vi "main_cr.vi"() -> ()   [LabVIEW 2017]
panel:
  out "error out 6":errorcluster
  in  "MoveL":bool
  out "error out 5":errorcluster
  out "error out 4":errorcluster
  out "error out 3":errorcluster
  out "DigitalOutput":u8[](array[numeric])
  out "DigitalInput":u8[](array[numeric])
  out "Current SpeedFactor":dbl
  out "error out 2":errorcluster
  in  "Digital Outputs Index:":i32=1 min=1 max=16 step=1
  out "Error Log":string
  in  "GetErrorID":bool
  out "x value":string
  out "y value":string
  out "z value":string
  out "rx value":string
  out "ry value":string
  out "rz value":string
  out "j6 value":string
  out "j5 value":string
  out "j4 value":string
  out "j3 value":string
  out "j2 value":string
  out "j1 value":string
  in  "rz-":bool
  in  "ry-":bool
  in  "rx-":bool
  in  "z-":bool
  in  "y-":bool
  in  "x-":bool
  in  "rz+":bool
  in  "ry+":bool
  in  "rx+":bool
  in  "z+":bool
  in  "y+":bool
  in  "x+":bool
  in  "JointMovJ":bool
  in  "j6":dbl
  in  "j5":dbl
  in  "j4":dbl
  in  "j3":dbl
  in  "j2":dbl
  in  "j1":dbl
  in  "Set IO confrim":bool
  in  "Status":string(combo)="1"
  in  "Reset Robot":bool
  in  "Feedback Port":string="30004"
  in  "Move Port":string="30003"
  in  "Dashboard Port":string="29999"
  in  "IP Address":string="192.168.5.1"
  in  "stop get state":bool
  out "state error out 2":errorcluster
  out "Robot mode":T1(ring)
  out "speed set string":string
  in  "j6-":bool
  in  "j5-":bool
  in  "j4-":bool
  in  "j3-":bool
  in  "j2-":bool
  in  "j1-":bool
  in  "j6+":bool
  in  "j5+":bool
  in  "j4+":bool
  in  "j3+":bool
  in  "j2+":bool
  in  "j1+":bool
  out "error out":errorcluster
  in  "stop connect":bool
  in  "Start trace":bool
  in  "tracePath":string
  in  "Stop move":bool
  in  "MoveJ":bool
  in  "rz":dbl
  in  "ry":dbl
  in  "rx":dbl
  in  "z":dbl
  in  "y":dbl
  in  "x":dbl
  in  "Speed confrim":bool
  in  "Speed Ratio":dbl=50.0
  in  "Emergency Stop":bool
  in  "Power up":bool
  out "Log":string
  in  "ClearError":bool
  in  "Enable Robot":bool
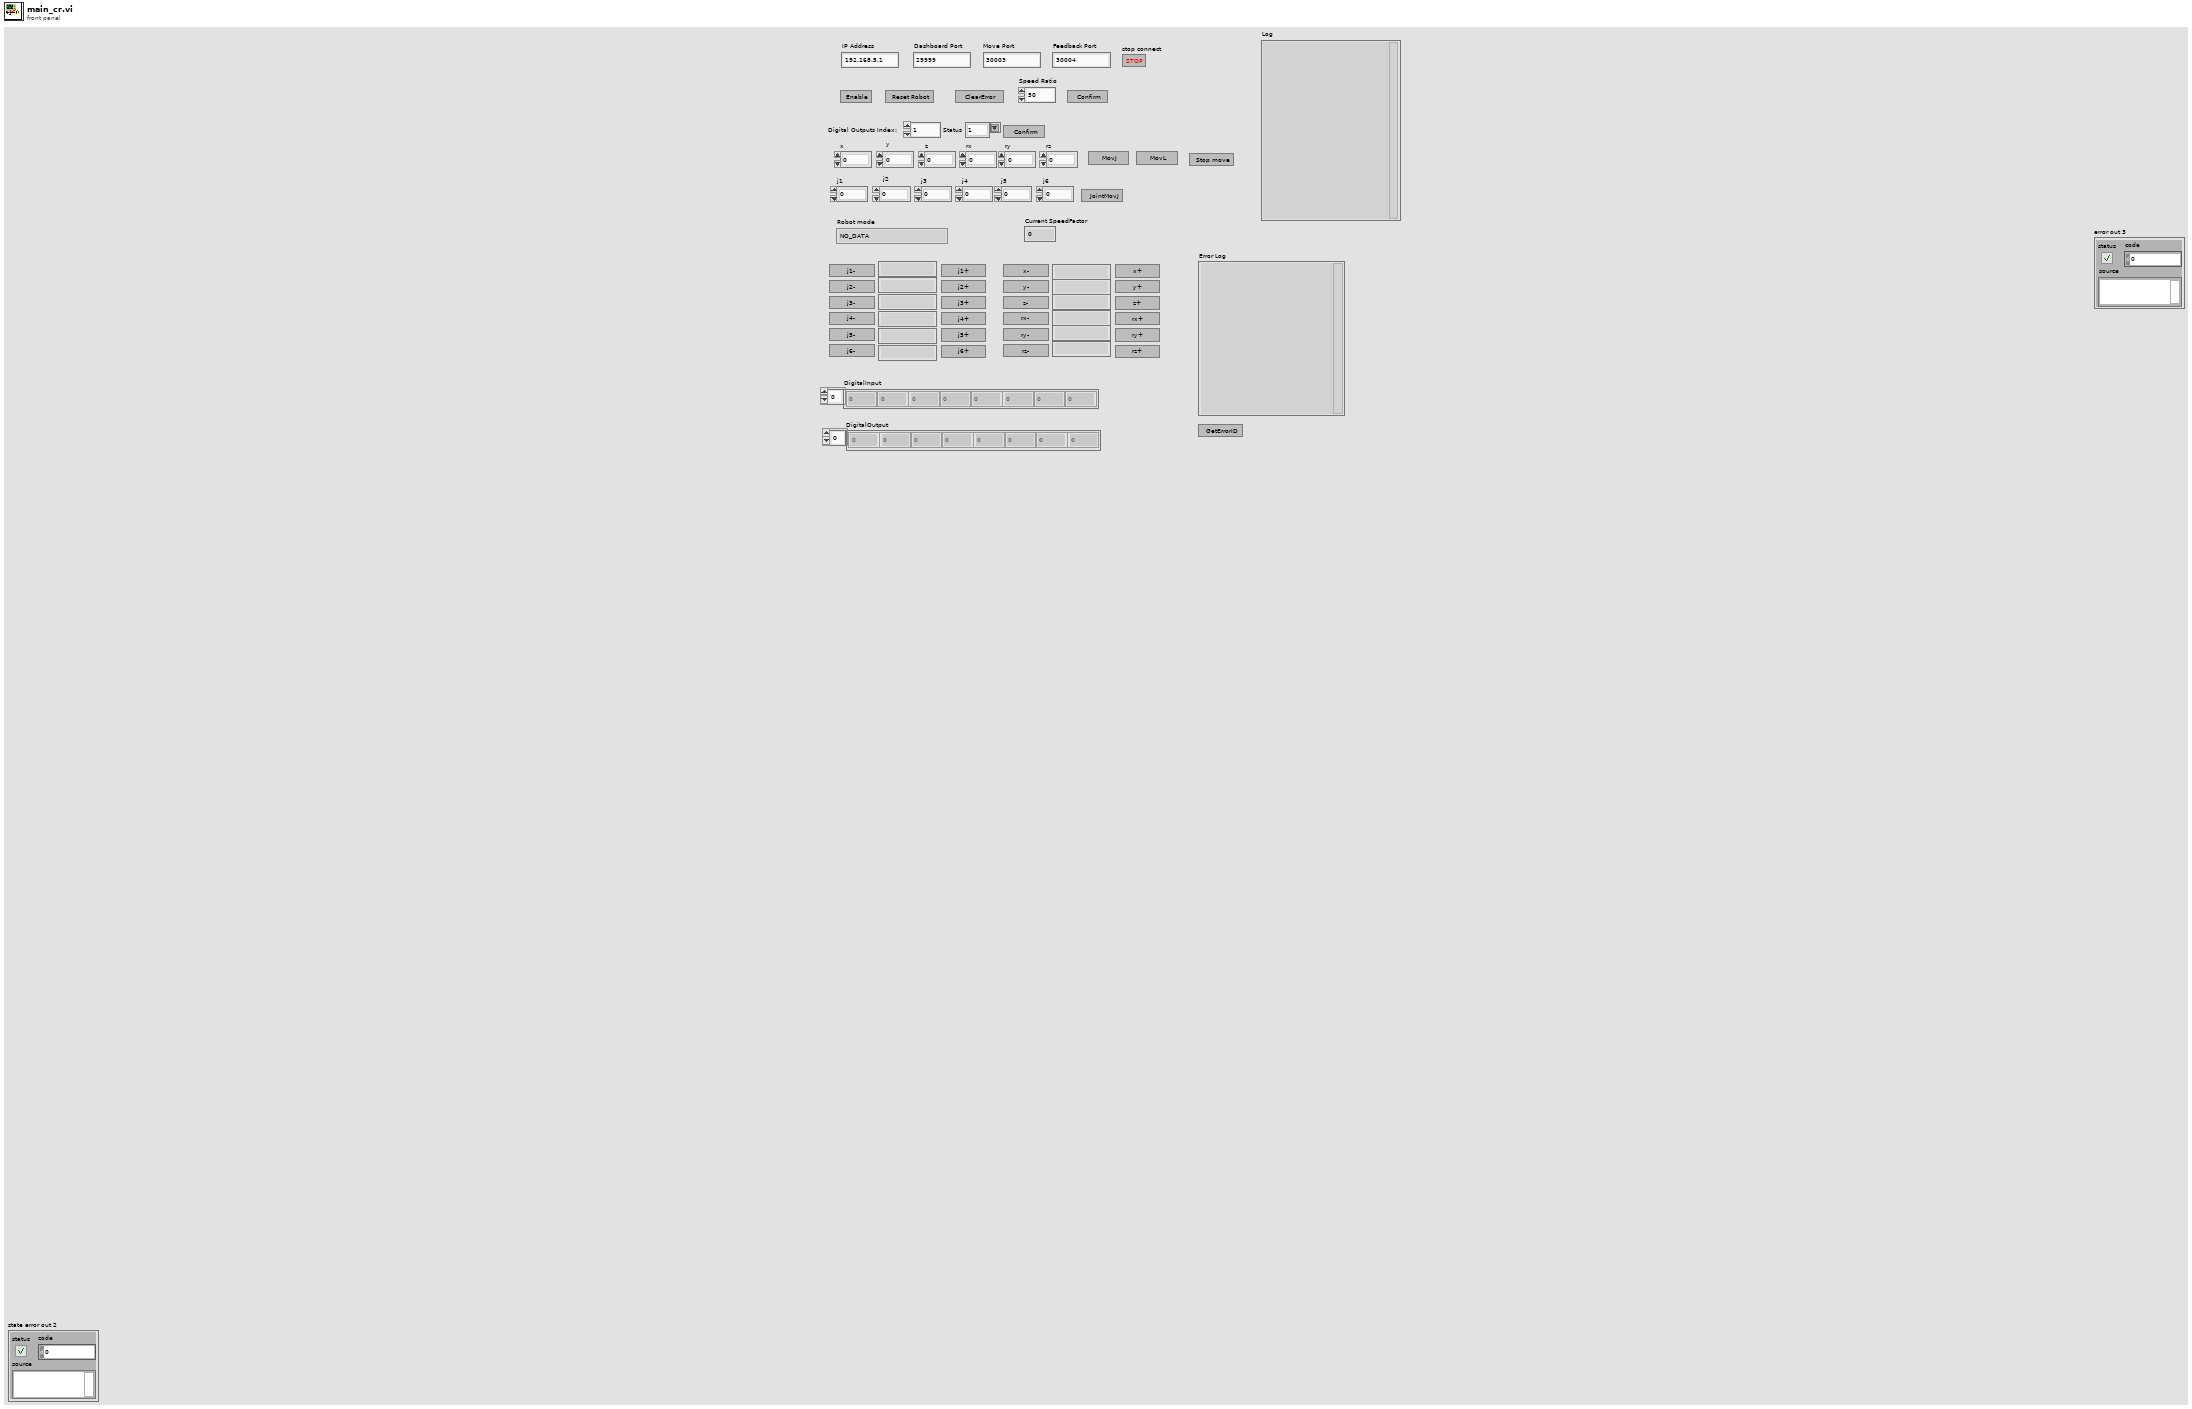
[diagram p1: front panel]
types:
  T1 = enum16{"NO_DATA", "ROBOT_MODE_INIT", "ROBOT_MODE_BRAKE_OPEN", "HOLD_BITS", "ROBOT_MODE_DISABLED", "ROBOT_MODE_ENABLE", "ROBOT_MODE_BACKDRIVE", "ROBOT_MODE_RUNNING", "ROBOT_MODE_RECORDING", "ROBOT_MODE_ERROR", "ROBOT_MODE_PAUSE", "ROBOT_MODE_JOG"}
  T2 = enum16{"Standard", "Buffered", "CRLF", "Immediate"}
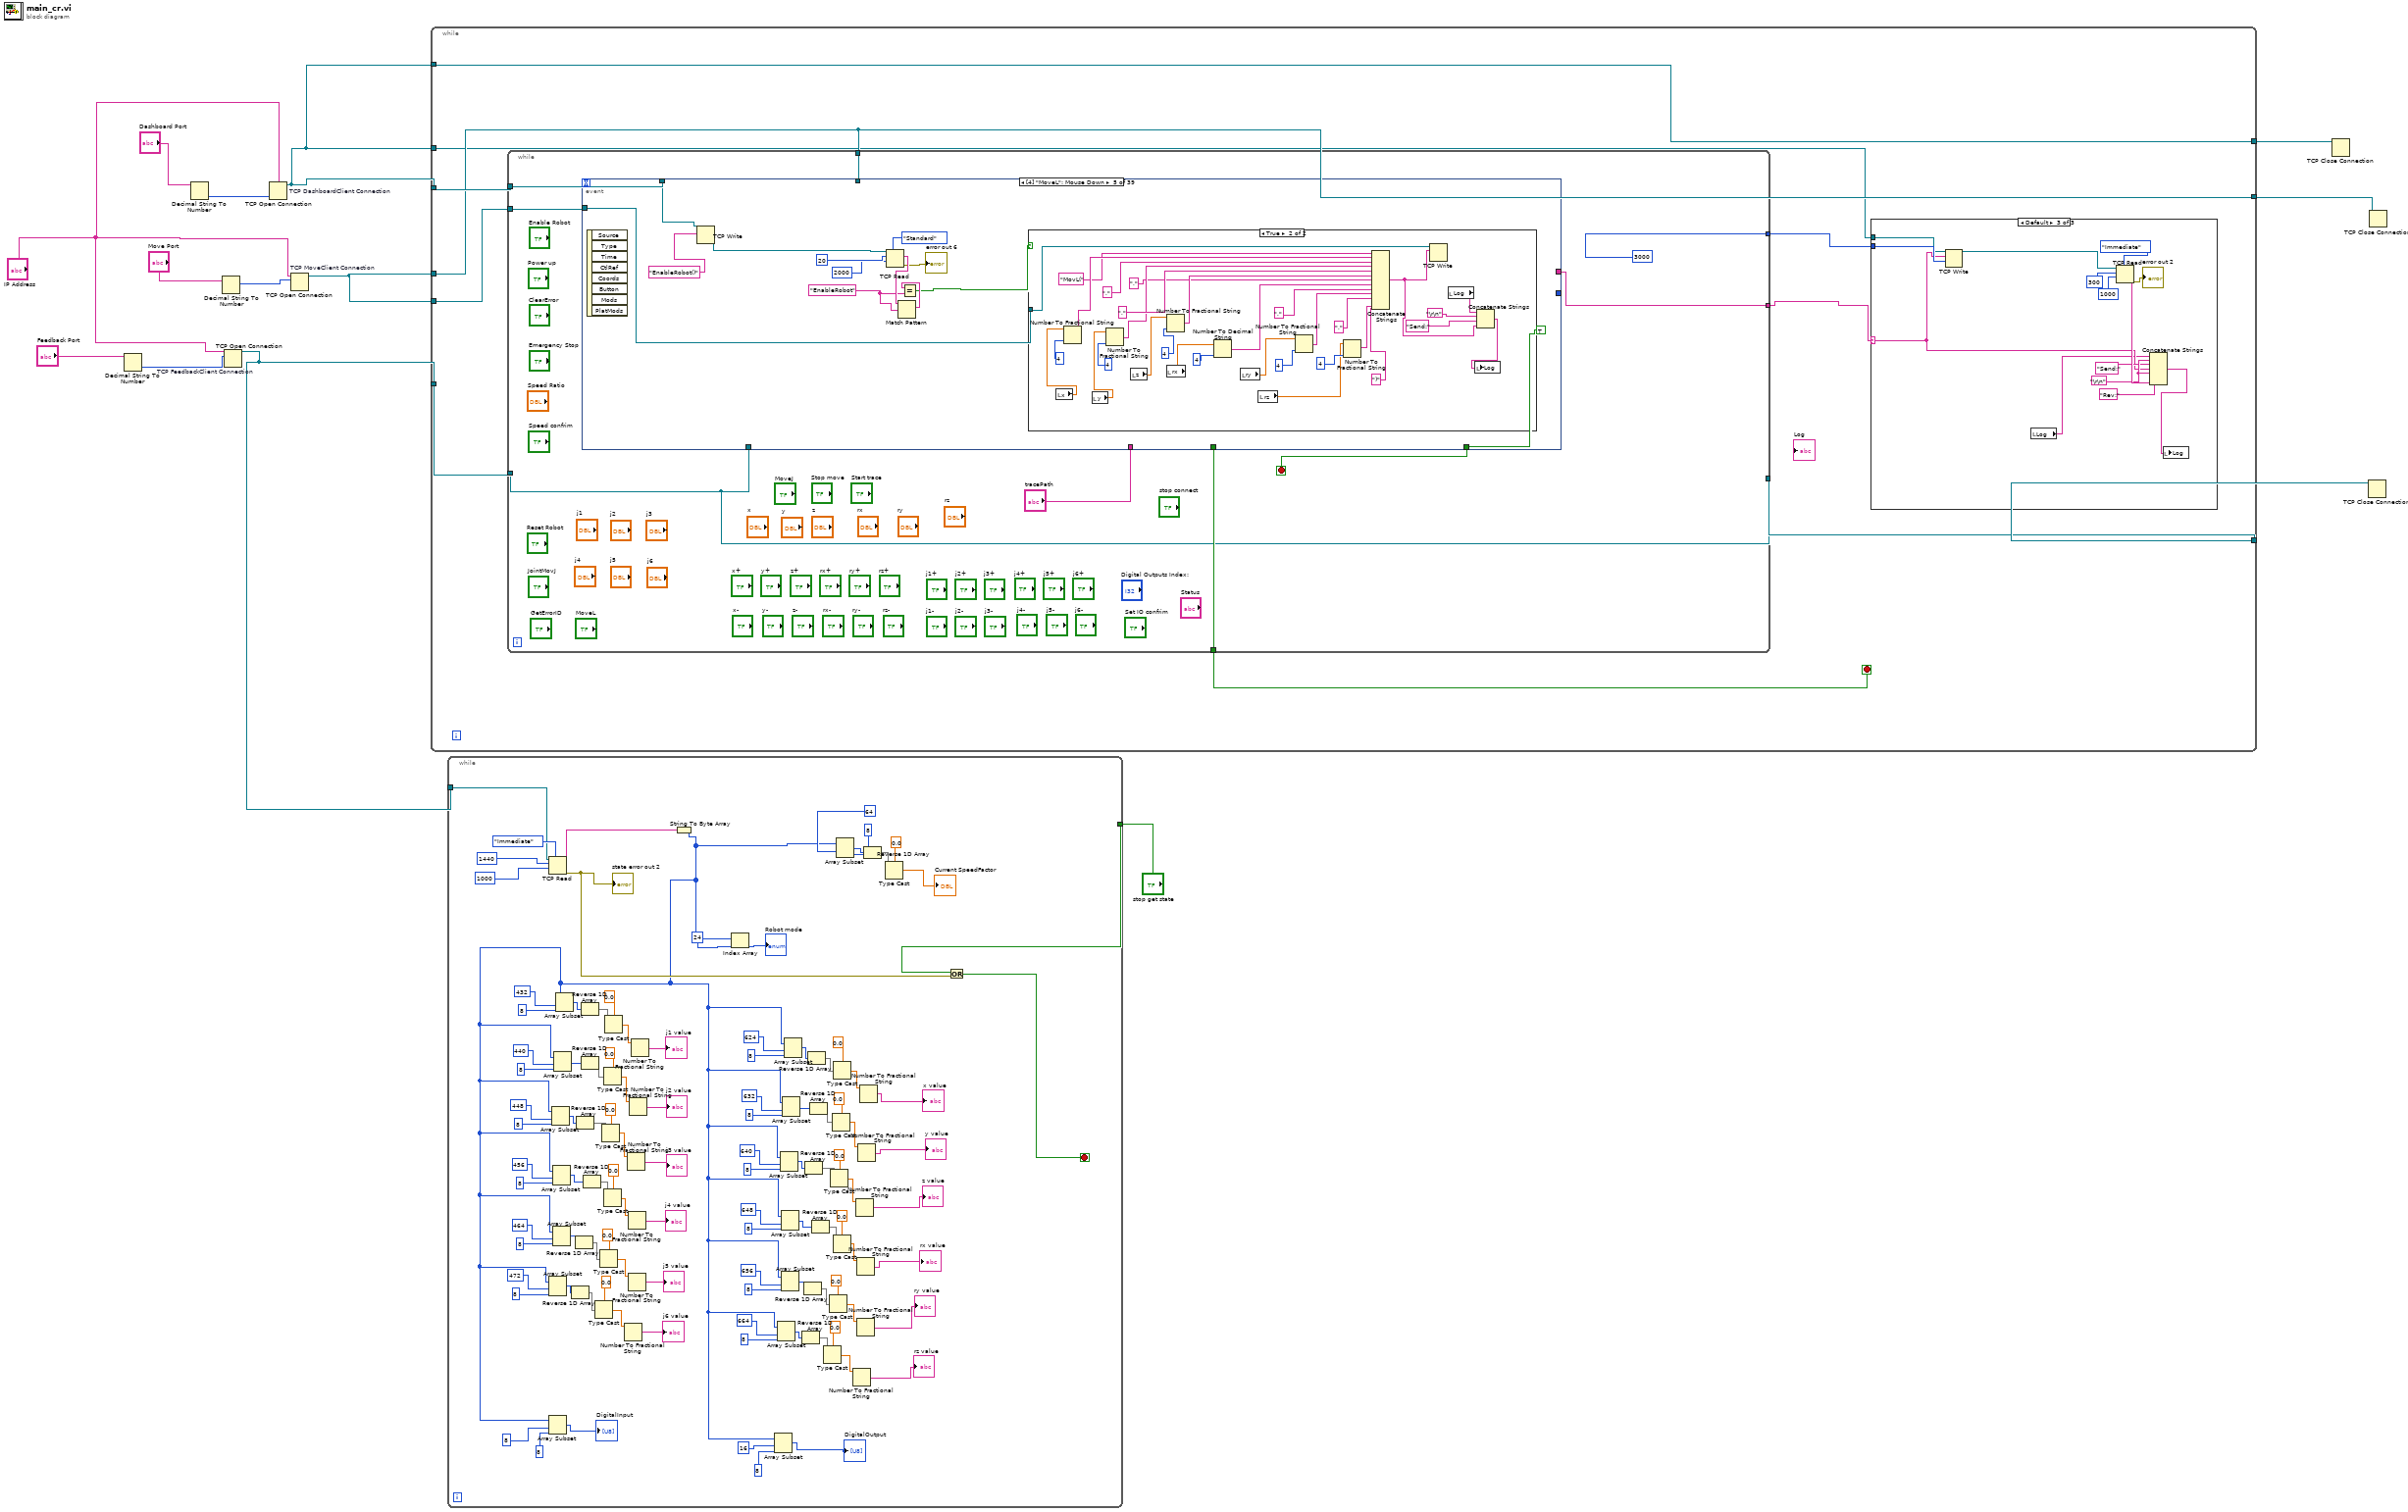
[diagram p0: block diagram]
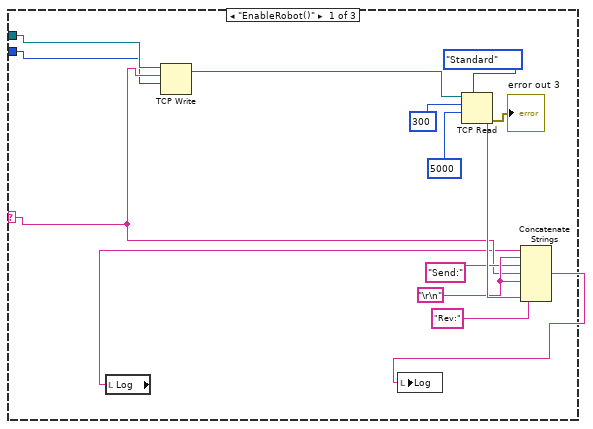
[diagram p2: hidden frame]
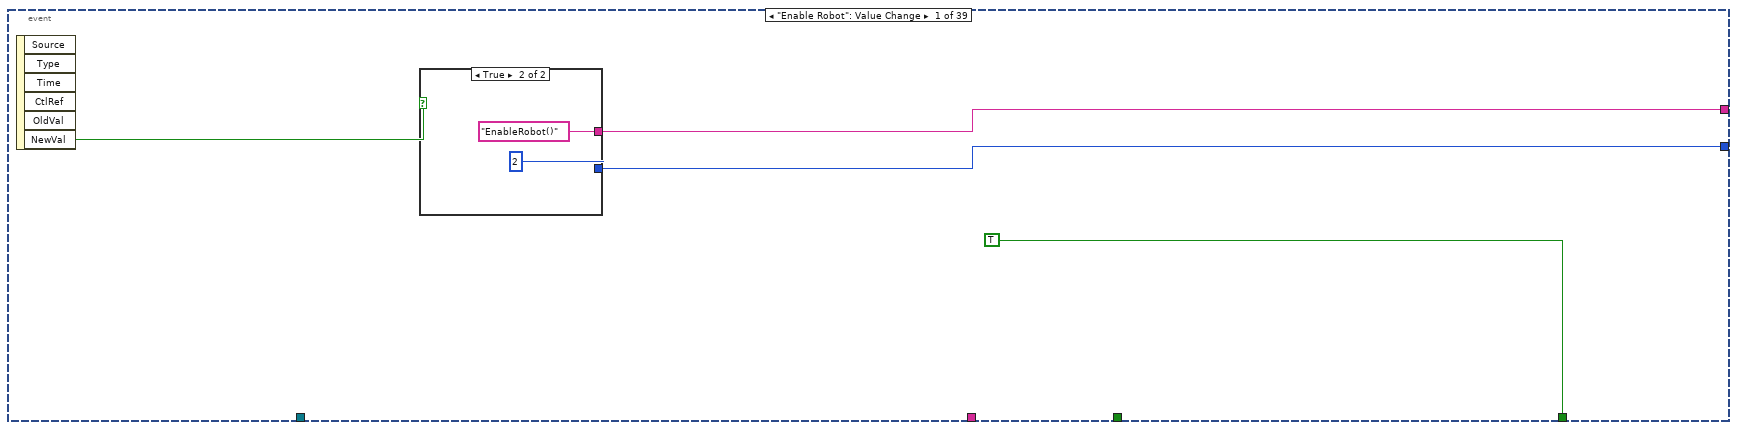
[diagram p4: hidden frame]
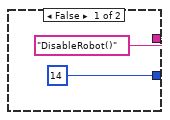
[diagram p5: hidden frame]
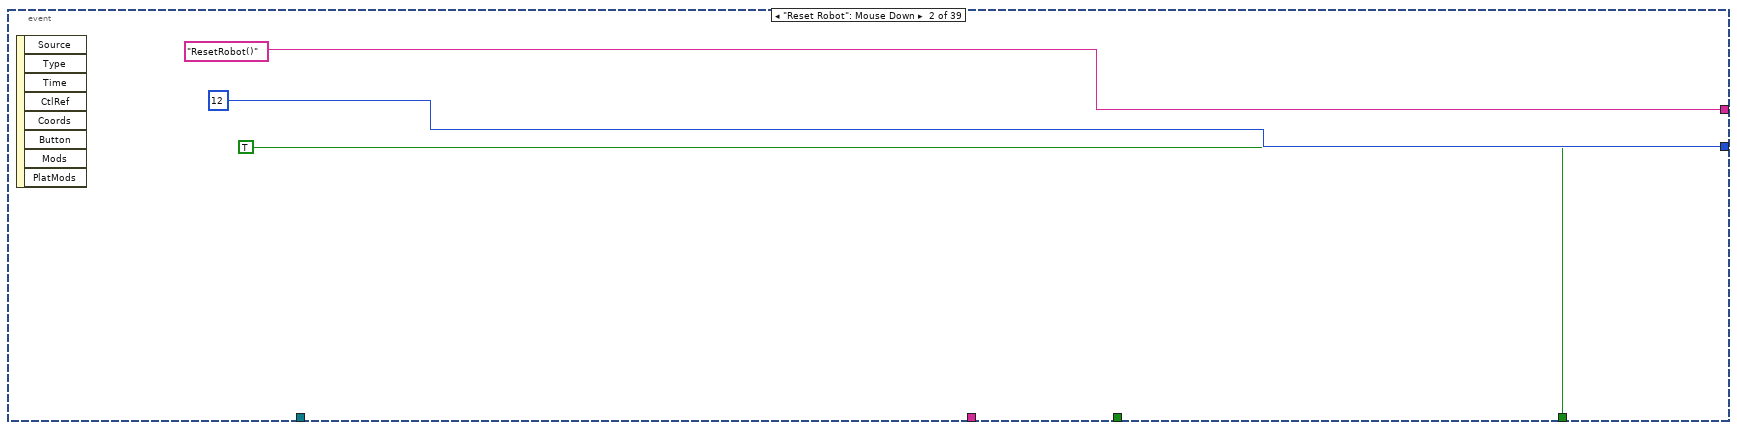
[diagram p6: hidden frame]
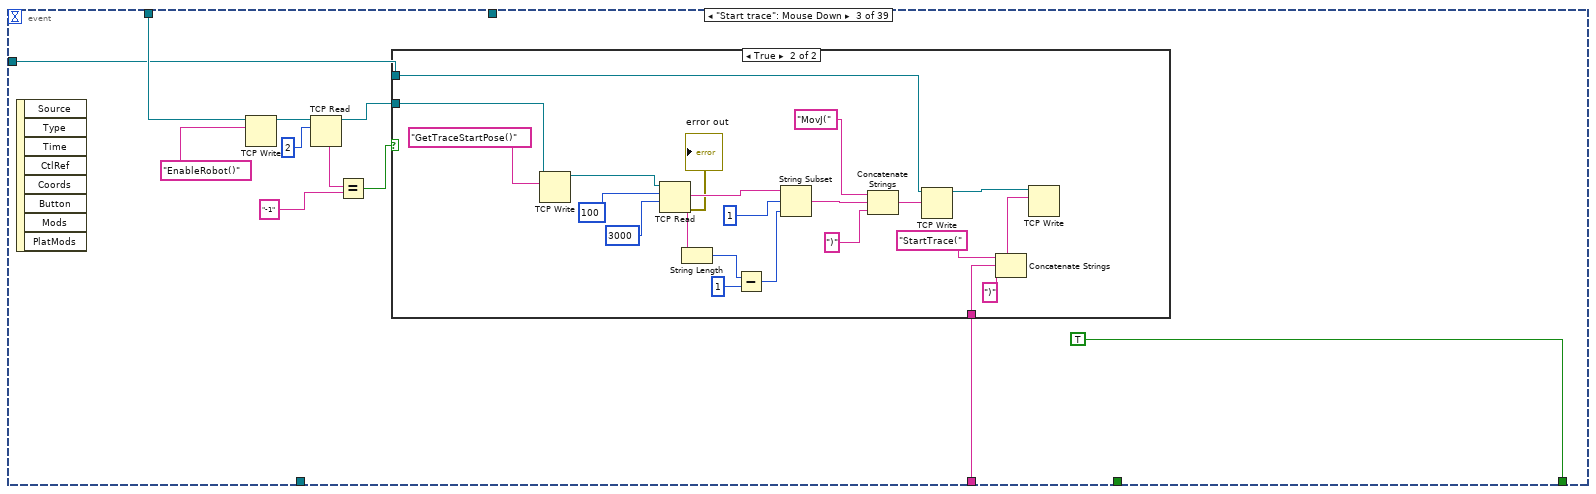
[diagram p7: hidden frame]
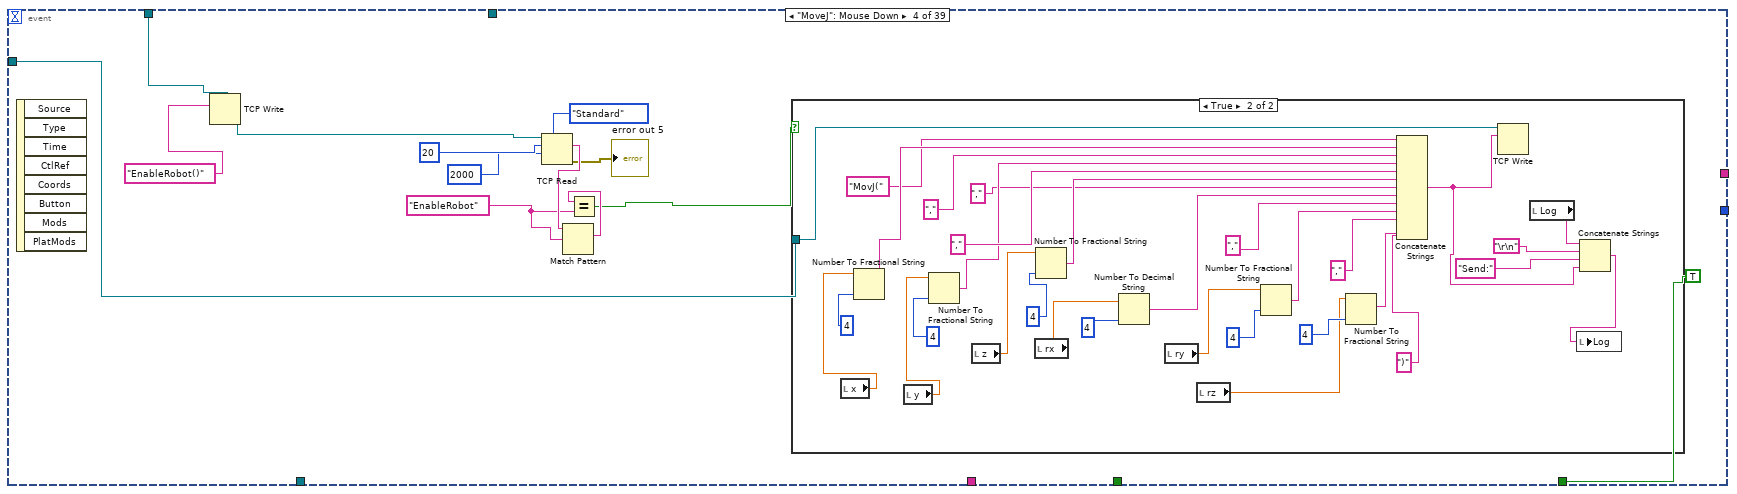
[diagram p9: hidden frame]
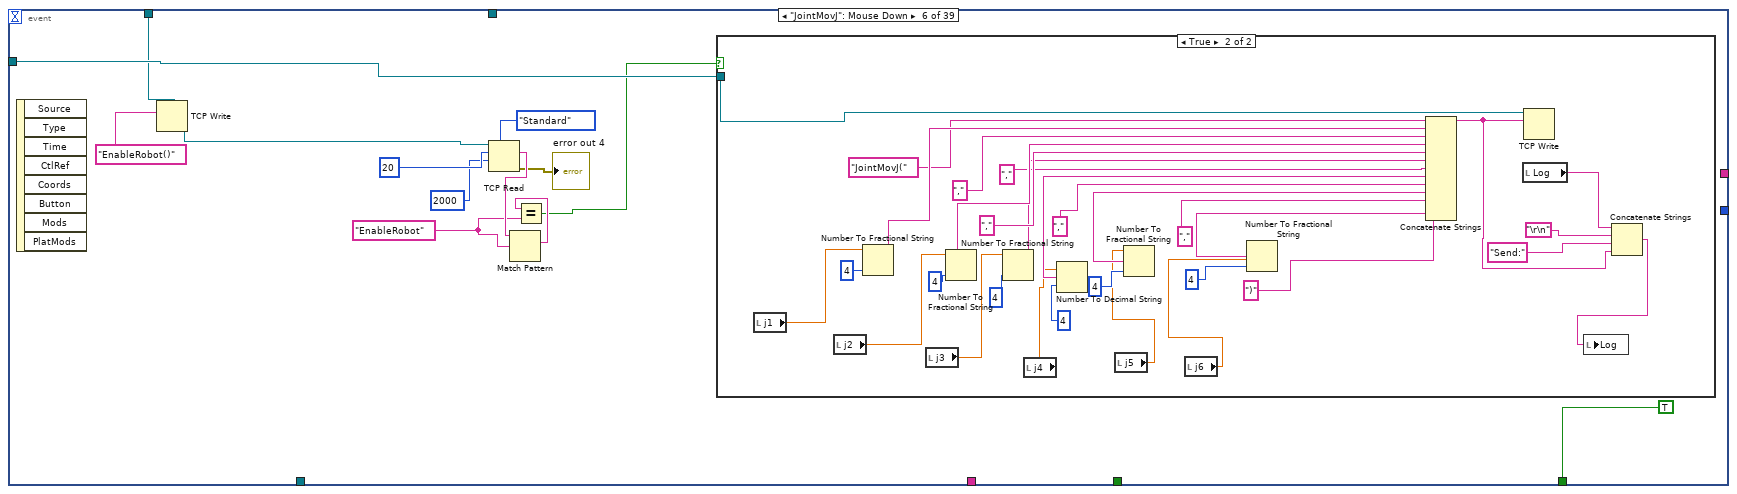
[diagram p12: hidden frame]
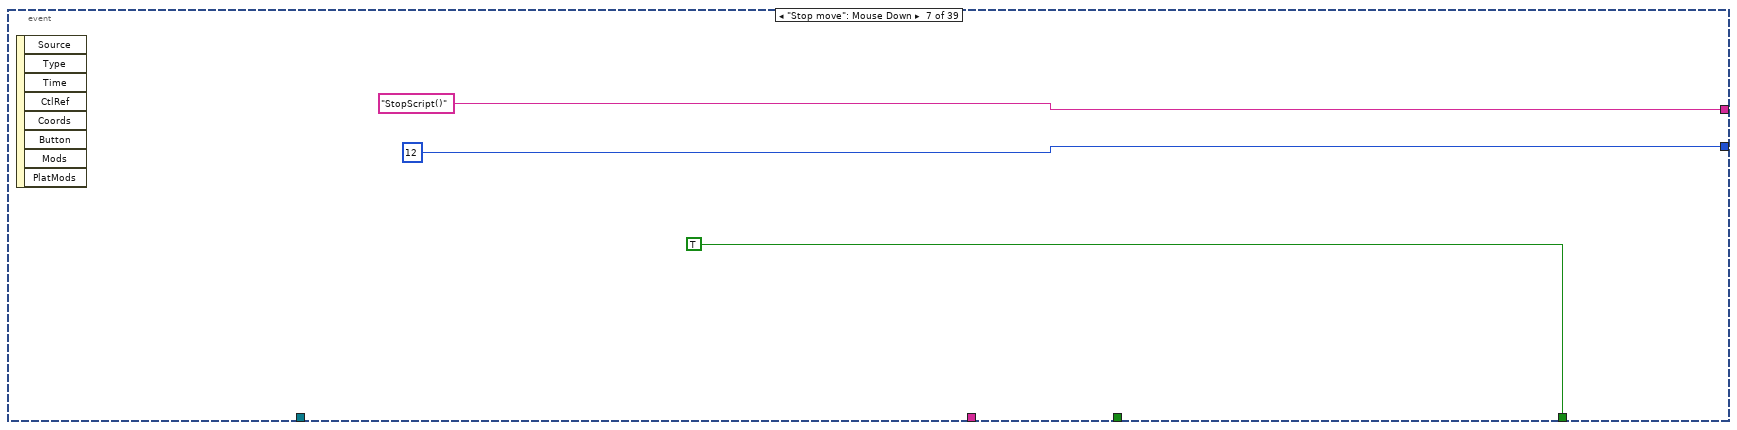
[diagram p14: hidden frame]
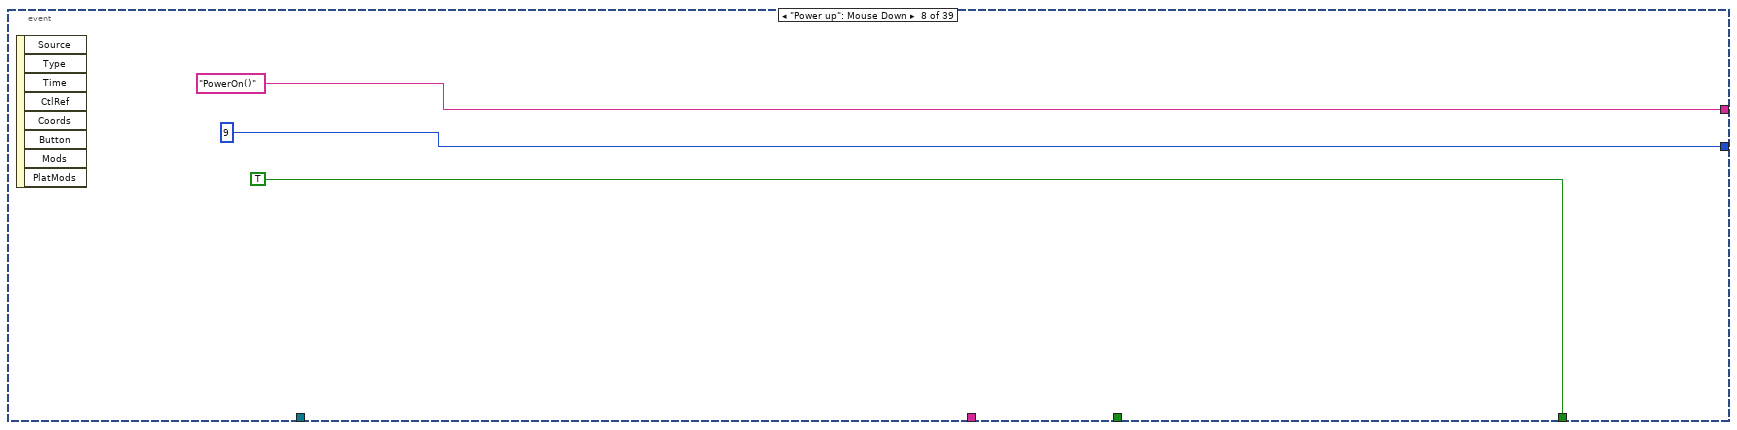
[diagram p15: hidden frame]
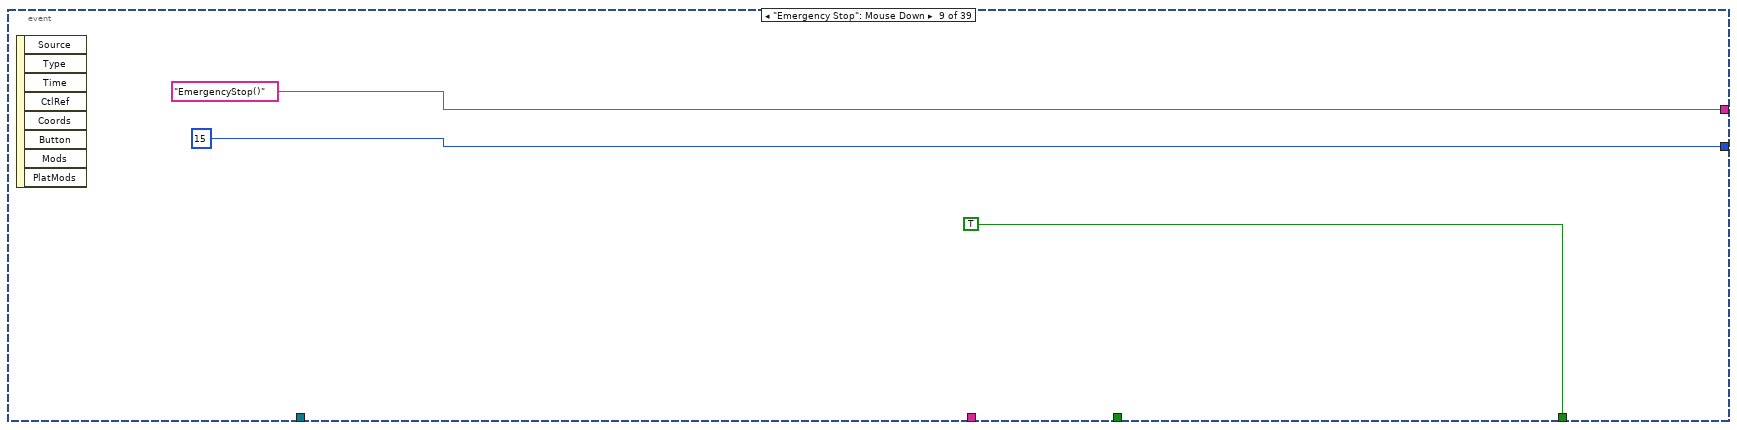
[diagram p16: hidden frame]
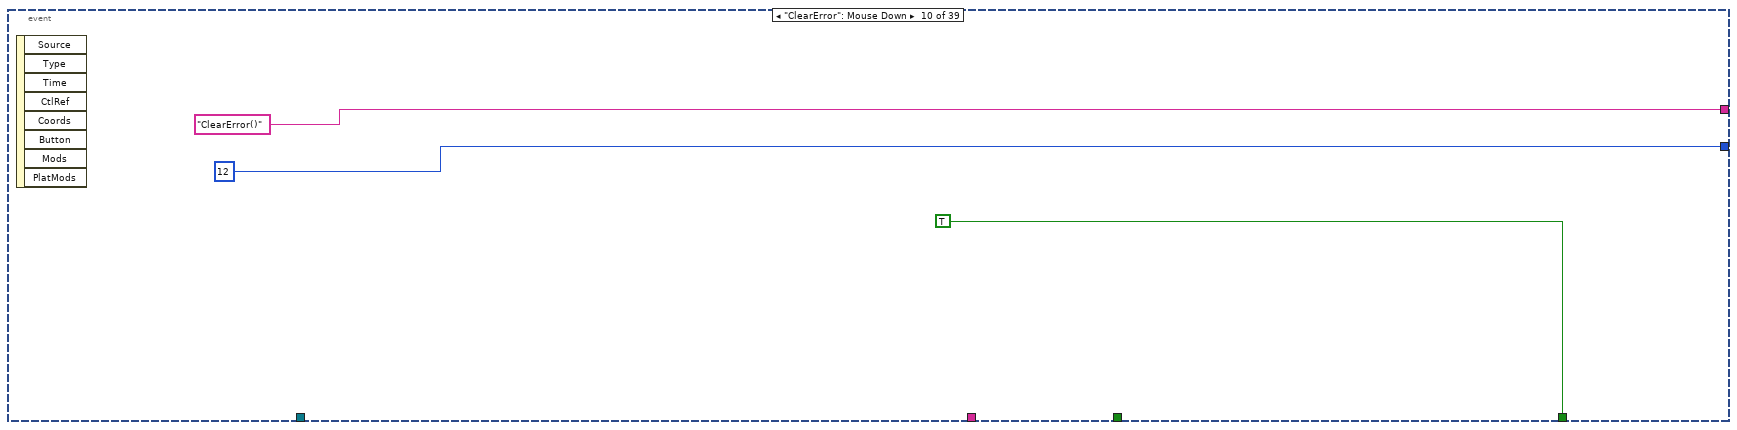
[diagram p17: hidden frame]
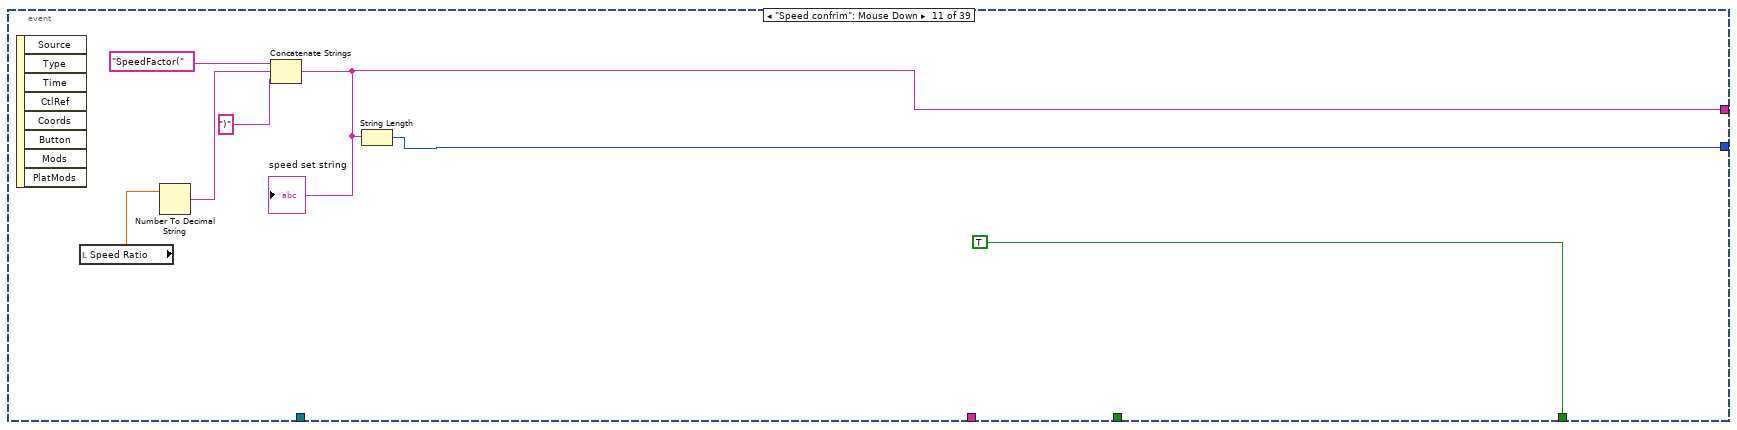
[diagram p18: hidden frame]
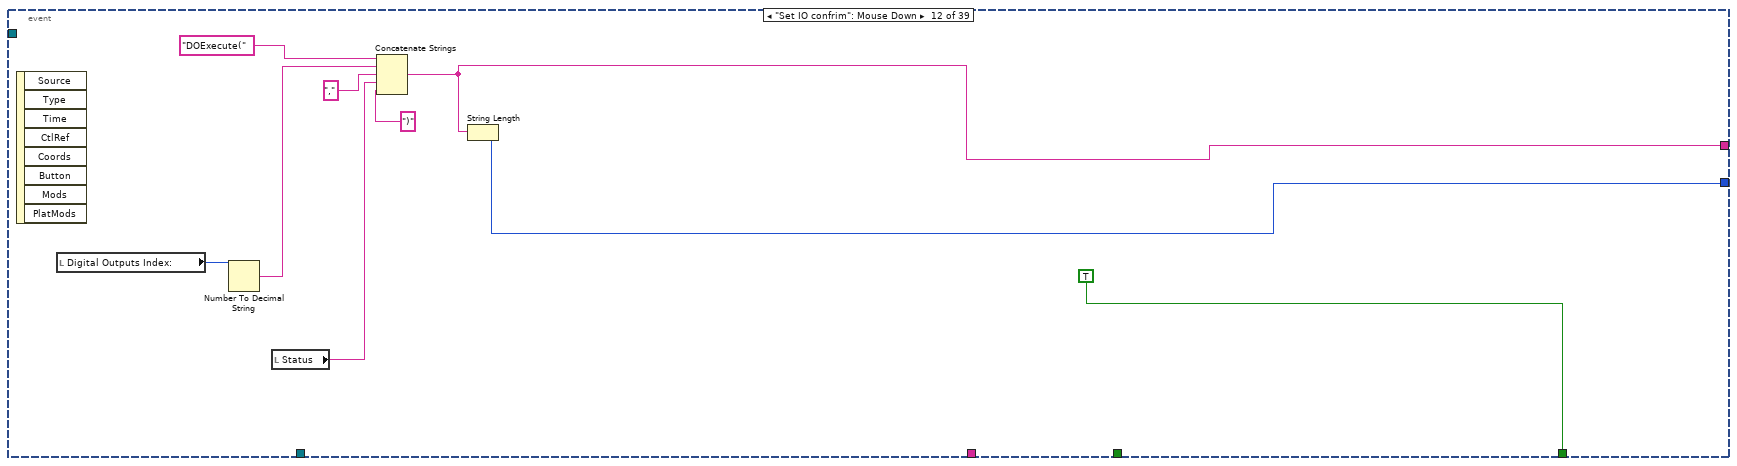
[diagram p19: hidden frame]
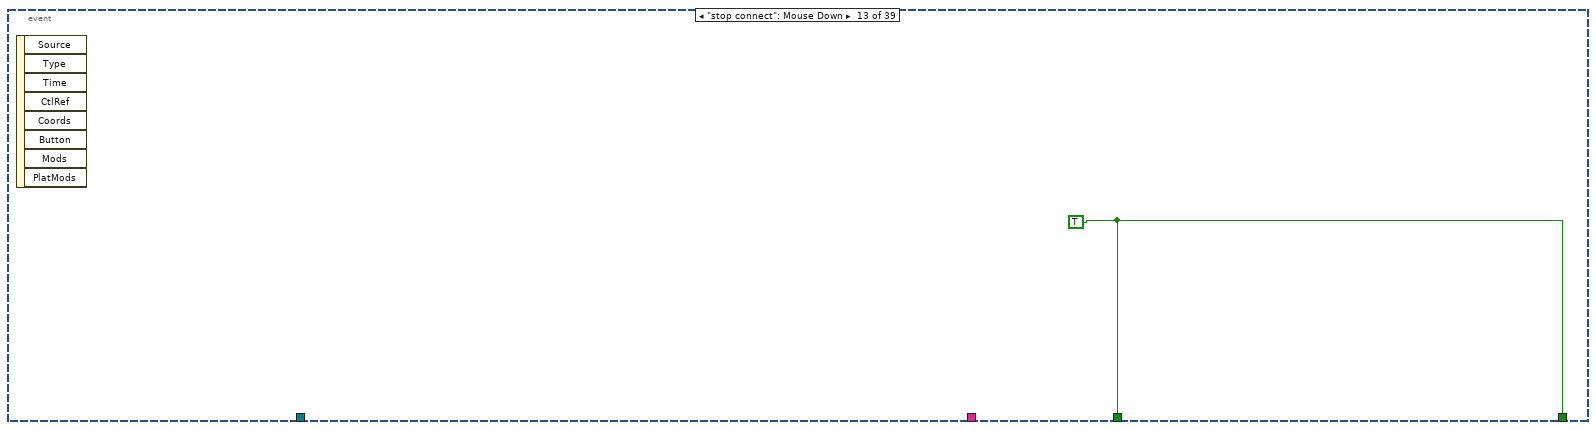
[diagram p20: hidden frame]
diagram:
  n1 = Decimal String To Number(string="Feedback Port") -> (number=w2:i32)  [unwired: 2 in, 1 out]
  n2 = Decimal String To Number(string="Dashboard Port") -> (number=w4:i32)  [unwired: 2 in, 1 out]
  n3 = Decimal String To Number(string="Move Port") -> (number=w3:i32)  [unwired: 2 in, 1 out]
  n4 = TCP Open Connection "TCP FeedbackClient Connection"(address="IP Address", remote port or service name=w2) -> (connection ID=w9:refnum<k5>)  [unwired: 3 in, 1 out]
  n5 = TCP Open Connection "TCP DashboardClient Connection"(address="IP Address", remote port or service name=w4) -> (connection ID=w1:refnum<k5>)  [unwired: 3 in, 1 out]
  n6 = TCP Open Connection "TCP MoveClient Connection"(address="IP Address", remote port or service name=w3) -> (connection ID=w12:refnum<k5>)  [unwired: 3 in, 1 out]
  n7 = while {
    tunnel: [w18] -> w14
    tunnel: w12 -> [w18]
    tunnel: [w24] -> w13
    tunnel: w1 -> [w24]
    tunnel: w1 -> [w23]
    tunnel: w12 -> [w22]
    tunnel: w9 -> [w20]
    tunnel: [w19] -> w11
    tunnel: w1 -> [w16]
    stop <- w21 stop-if-true
    n8 = while {
      tunnel: w23 -> [w61]
      tunnel: w22 -> [w60]
      tunnel: [w57] -> w21
      tunnel: w20 -> [w56]
      tunnel: [w56] -> w19
      tunnel: w18 -> [w55]
      tunnel: [w54] -> w15
      tunnel: [3000 ("timeout ms (25000)")] -> w17
      stop <- w58 stop-if-true
      n9 = event shown="[4] \"MoveL\": Mouse Down" {
        selector: _ -> [_ _ _ _ _ _ _ _ _ _ _ _ _ _ _ _ _ _ _ _ _ _ _ _ _ _ _ _ _ _ _ _ _ _ _ _ _ _ _]
        dyn-events: _ -> [_ _ _ _ _ _ _ _ _ _ _ _ _ _ _ _ _ _ _ _ _ _ _ _ _ _ _ _ _ _ _ _ _ _ _ _ _ _ _]
        timeout: _ -> [_ _ _ _ _ _ _ _ _ _ _ _ _ _ _ _ _ _ _ _ _ _ _ _ _ _ _ _ _ _ _ _ _ _ _ _ _ _ _]
        tunnel: [w62 "ResetRobot()" _ _ _ _ "StopScript()" "PowerOn()" "EmergencyStop()" "ClearError()" w250 w259 _ _ _ _ _ _ _ _ _ _ _ _ _ _ _ _ _ _ _ _ _ _ _ _ _ _ _] -> w54
        tunnel: [w64 12 _ _ _ _ 12 9 15 12 w253 w260 _ _ _ _ _ _ _ _ _ _ _ _ _ _ _ _ _ _ _ _ _ _ _ _ _ _ _] -> _
        tunnel: w61 -> [_ _ w78 w109 w153 w197 _ _ _ _ _ _ _ _ _ _ _ _ _ _ _ _ _ _ _ _ _ _ _ _ _ _ _ _ _ _ _ _ _]
        tunnel: w60 -> [_ _ w75 w117 w161 w204 _ _ _ _ _ _ _ _ w274 w276 w278 w280 w282 w284 w286 w288 w290 w292 w294 w296 w298 w300 w302 w304 w306 w308 w310 w312 w314 w316 w318 w320 w322]
        tunnel: "tracePath" -> [_ _ w74 _ _ _ _ _ _ _ _ _ _ _ _ _ _ _ _ _ _ _ _ _ _ _ _ _ _ _ _ _ _ _ _ _ _ _ _]
        tunnel: [TRUE TRUE TRUE TRUE TRUE TRUE TRUE TRUE TRUE TRUE TRUE TRUE w265 TRUE _ _ _ _ _ _ _ _ _ _ _ _ _ _ _ _ _ _ _ _ _ _ _ _ _] -> w58
        tunnel: [_ _ _ _ _ _ _ _ _ _ _ _ w265 _ _ _ _ _ _ _ _ _ _ _ _ _ _ _ _ _ _ _ _ _ _ _ _ _ _] -> w57
        tunnel: w56 -> [_ _ _ _ _ _ _ _ _ _ _ _ _ _ _ _ _ _ _ _ _ _ _ _ _ _ _ _ _ _ _ _ _ _ _ _ _ _ _]
        tunnel: w55 -> [_ _ _ _ _ _ _ _ _ _ _ _ _ w271 _ _ _ _ _ _ _ _ _ _ _ _ _ _ _ _ _ _ _ _ _ _ _ _ _]
        event "Enable Robot": Value Change {
          n10 = event-data() -> ("NewVal"=w65:bool)  [unwired: 1 in, 5 out]
          n11 = case shown="True" w65 {
            tunnel: ["DisableRobot()" "EnableRobot()"] -> w62
            tunnel: [14 2] -> w64
            frame False {
            }
            frame True {
            }
          }
        }
        event "Reset Robot": Mouse Down {
          n12 = event-data() -> ()  [unwired: 1 in, 8 out]
        }
        event "Start trace": Mouse Down {
          n13 = event-data() -> ()  [unwired: 1 in, 8 out]
          n14 = TCP Write(connection ID=w78, data in="EnableRobot()") -> (connection ID out=w83:refnum<k5>)  [unwired: 2 in, 2 out]
          n15 = TCP Read(connection ID=w83, bytes to read=2) -> (connection ID out=w76:refnum<k5>, data out=w80:string)  [unwired: 3 in, 1 out]
          n16 = Equal?(x=w80, y="-1") -> (x = y?=w77:bool)
          n17 = case shown="True" w77 {
            tunnel: w76 -> [_ w103]
            tunnel: w75 -> [_ w90]
            tunnel: w74 -> [_ w86]
            frame False {
            }
            frame True {
              n18 = TCP Write(connection ID=w103, data in="GetTraceStartPose()") -> (connection ID out=w101:refnum<k5>)  [unwired: 2 in, 2 out]
              n19 = TCP Read(connection ID=w101, bytes to read=100, 9:3000 ("timeout ms (25000)")) -> (data out=w98:string, error out=→"error out":errorcluster)  [unwired: 2 in, 1 out]
              n20 = String Length(string=w98) -> (length=w97:i32)
              n21 = Subtract(x=w97, y=1) -> (x-y=w95:i32)
              n22 = String Subset(string=w98, offset (0)=1, length (rest)=w95) -> (substring=w93:string)
              n23 = Concatenate Strings("MovJ(" ("string"), w93, ")" ("string")) -> (w91:string)
              n24 = TCP Write(connection ID=w90, data in=w91) -> (connection ID out=w89:refnum<k5>)  [unwired: 2 in, 2 out]
              n25 = Concatenate Strings("StartTrace(" ("string"), w86, ")" ("string")) -> (w87:string)
              n26 = TCP Write(connection ID=w89, data in=w87) -> ()  [unwired: 2 in, 3 out]
            }
          }
        }
        event "MoveJ": Mouse Down {
          w112 = "EnableRobot" ("y")
          n27 = event-data() -> ()  [unwired: 1 in, 8 out]
          n28 = TCP Write(connection ID=w109, data in="EnableRobot()") -> (connection ID out=w115:refnum<k5>)  [unwired: 2 in, 2 out]
          n29 = TCP Read(connection ID=w115, bytes to read=20, 7:T2."Standard" ("mode (standard)"), 9:2000 ("timeout ms (25000)")) -> (data out=w114:string, error out=→"error out 5":errorcluster)  [unwired: 1 in, 1 out]
          n30 = Match Pattern(string=w114, regular expression=w112) -> (match substring=w113:string)  [unwired: 1 in, 3 out]
          n31 = Equal?(x=w113, y=w112) -> (x = y?=w107:bool)
          n32 = case shown="True" w107 {
            tunnel: w117 -> [_ w148]
            frame False {
            }
            frame True {
              n33 = local read "x"() -> (w123:dbl)
              n34 = Number To Fractional String(number=w123, precision (6)=i16 4) -> (F-format string=w147:string)  [unwired: 2 in]
              n35 = local read "y"() -> (w124:dbl)
              n36 = Number To Fractional String(number=w124, precision (6)=i16 4) -> (F-format string=w143:string)  [unwired: 2 in]
              n37 = local read "z"() -> (w125:dbl)
              n38 = local read "rx"() -> (w126:dbl)
              n39 = Number To Fractional String(number=w125, precision (6)=i16 4) -> (F-format string=w133:string)  [unwired: 2 in]
              n40 = Number To Decimal String(number=w126, width (-)=i16 4 ("precision (6)")) -> (decimal integer string=w142:string)
              n41 = local read "ry"() -> (w127:dbl)
              n42 = local read "rz"() -> (w128:dbl)
              n43 = Number To Fractional String(number=w127, precision (6)=i16 4) -> (F-format string=w140:string)  [unwired: 2 in]
              n44 = Number To Fractional String(number=w128, precision (6)=i16 4) -> (F-format string=w138:string)  [unwired: 2 in]
              n45 = Concatenate Strings("MovJ(" ("string"), w147, "," ("string"), w143, "," ("string"), w133, "," ("string"), w142, "," ("string"), w140, "," ("string"), w138, ")" ("string")) -> (w119:string)
              n46 = TCP Write(connection ID=w148, data in=w119) -> ()  [unwired: 2 in, 3 out]
              n47 = local read "Log"() -> (w122:string)
              n48 = Concatenate Strings(w122, "\r\n", "Send:" ("string"), w119) -> (w118:string)
              n49 = local write "Log"(w118) -> ()
            }
          }
        }
        event "MoveL": Mouse Down {
          w156 = "EnableRobot" ("y")
          n50 = event-data() -> ()  [unwired: 1 in, 8 out]
          n51 = TCP Write(connection ID=w153, data in="EnableRobot()") -> (connection ID out=w159:refnum<k5>)  [unwired: 2 in, 2 out]
          n52 = TCP Read(connection ID=w159, bytes to read=20, 7:T2."Standard" ("mode (standard)"), 9:2000 ("timeout ms (25000)")) -> (data out=w158:string, error out=→"error out 6":errorcluster)  [unwired: 1 in, 1 out]
          n53 = Match Pattern(string=w158, regular expression=w156) -> (match substring=w157:string)  [unwired: 1 in, 3 out]
          n54 = Equal?(x=w157, y=w156) -> (x = y?=w151:bool)
          n55 = case shown="True" w151 {
            tunnel: w161 -> [_ w192]
            frame False {
            }
            frame True {
              n56 = local read "x"() -> (w167:dbl)
              n57 = Number To Fractional String(number=w167, precision (6)=i16 4) -> (F-format string=w191:string)  [unwired: 2 in]
              n58 = local read "y"() -> (w168:dbl)
              n59 = Number To Fractional String(number=w168, precision (6)=i16 4) -> (F-format string=w187:string)  [unwired: 2 in]
              n60 = local read "z"() -> (w169:dbl)
              n61 = local read "rx"() -> (w170:dbl)
              n62 = Number To Fractional String(number=w169, precision (6)=i16 4) -> (F-format string=w177:string)  [unwired: 2 in]
              n63 = Number To Decimal String(number=w170, width (-)=i16 4 ("precision (6)")) -> (decimal integer string=w186:string)
              n64 = local read "ry"() -> (w171:dbl)
              n65 = local read "rz"() -> (w172:dbl)
              n66 = Number To Fractional String(number=w171, precision (6)=i16 4) -> (F-format string=w184:string)  [unwired: 2 in]
              n67 = Number To Fractional String(number=w172, precision (6)=i16 4) -> (F-format string=w182:string)  [unwired: 2 in]
              n68 = Concatenate Strings("MovL(" ("string"), w191, "," ("string"), w187, "," ("string"), w177, "," ("string"), w186, "," ("string"), w184, "," ("string"), w182, ")" ("string")) -> (w163:string)
              n69 = TCP Write(connection ID=w192, data in=w163) -> ()  [unwired: 2 in, 3 out]
              n70 = local read "Log"() -> (w166:string)
              n71 = Concatenate Strings(w166, "\r\n", "Send:" ("string"), w163) -> (w162:string)
              n72 = local write "Log"(w162) -> ()
            }
          }
        }
        event "JointMovJ": Mouse Down {
          w199 = "EnableRobot" ("y")
          n73 = event-data() -> ()  [unwired: 1 in, 8 out]
          n74 = TCP Write(connection ID=w197, data in="EnableRobot()") -> (connection ID out=w203:refnum<k5>)  [unwired: 2 in, 2 out]
          n75 = TCP Read(connection ID=w203, bytes to read=20, 7:T2."Standard" ("mode (standard)"), 9:2000 ("timeout ms (25000)")) -> (data out=w201:string, error out=→"error out 4":errorcluster)  [unwired: 1 in, 1 out]
          n76 = Match Pattern(string=w201, regular expression=w199) -> (match substring=w200:string)  [unwired: 1 in, 3 out]
          n77 = Equal?(x=w200, y=w199) -> (x = y?=w198:bool)
          n78 = case shown="True" w198 {
            tunnel: w204 -> [_ w236]
            frame False {
            }
            frame True {
              n79 = local read "j1"() -> (w213:dbl)
              n80 = local read "j2"() -> (w211:dbl)
              n81 = Number To Fractional String(number=w213, precision (6)=i16 4) -> (F-format string=w235:string)  [unwired: 2 in]
              n82 = local read "j3"() -> (w212:dbl)
              n83 = Number To Fractional String(number=w211, precision (6)=i16 4) -> (F-format string=w231:string)  [unwired: 2 in]
              n84 = Number To Fractional String(number=w212, precision (6)=i16 4) -> (F-format string=w221:string)  [unwired: 2 in]
              n85 = local read "j4"() -> (w214:dbl)
              n86 = Number To Decimal String(number=w214, width (-)=i16 4 ("precision (6)")) -> (decimal integer string=w230:string)
              n87 = local read "j5"() -> (w215:dbl)
              n88 = Number To Fractional String(number=w215, precision (6)=i16 4) -> (F-format string=w228:string)  [unwired: 2 in]
              n89 = local read "j6"() -> (w216:dbl)
              n90 = Number To Fractional String(number=w216, precision (6)=i16 4) -> (F-format string=w226:string)  [unwired: 2 in]
              n91 = Concatenate Strings("JointMovJ(" ("string"), w235, "," ("string"), w231, "," ("string"), w221, "," ("string"), w230, "," ("string"), w228, "," ("string"), w226, ")" ("string")) -> (w208:string)
              n92 = local read "Log"() -> (w207:string)
              n93 = TCP Write(connection ID=w236, data in=w208) -> ()  [unwired: 2 in, 3 out]
              n94 = Concatenate Strings(w207, "\r\n", "Send:" ("string"), w208) -> (w206:string)
              n95 = local write "Log"(w206) -> ()
            }
          }
        }
        event "Stop move": Mouse Down {
          n96 = event-data() -> ()  [unwired: 1 in, 8 out]
        }
        event "Power up": Mouse Down {
          n97 = event-data() -> ()  [unwired: 1 in, 8 out]
        }
        event "Emergency Stop": Mouse Down {
          n98 = event-data() -> ()  [unwired: 1 in, 8 out]
        }
        event "ClearError": Mouse Down {
          n99 = event-data() -> ()  [unwired: 1 in, 8 out]
        }
        event "Speed confrim": Mouse Down {
          n100 = event-data() -> ()  [unwired: 1 in, 8 out]
          n101 = local read "Speed Ratio"() -> (w249:dbl)
          n102 = Number To Decimal String(number=w249) -> (decimal integer string=w255:string)  [unwired: 1 in]
          n103 = Concatenate Strings("SpeedFactor(", w255, ")") -> (w250:string)
          "speed set string" <- w250
          n104 = String Length(string=w250) -> (length=w253:i32)
        }
        event "Set IO confrim": Mouse Down {
          n105 = event-data() -> ()  [unwired: 1 in, 8 out]
          n106 = local read "Digital Outputs Index:"() -> (w257:i32)
          n107 = Number To Decimal String(number=w257) -> (decimal integer string=w264:string)  [unwired: 1 in]
          n108 = local read "Status"() -> (w256:string)
          n109 = Concatenate Strings("DOExecute(", w264, "," ("string"), w256, ")") -> (w259:string)
          n110 = String Length(string=w259) -> (length=w260:i32)
        }
        event "stop connect": Mouse Down {
          w265 = TRUE
          n111 = event-data() -> ()  [unwired: 1 in, 8 out]
        }
        event "GetErrorID": Mouse Down {
          w269 = 3000 ("timeout ms (25000)")
          n112 = event-data() -> ()  [unwired: 1 in, 8 out]
          n113 = TCP Write(connection ID=w271, data in="GetErrorID()", 9:w269) -> (connection ID out=w270:refnum<k5>)  [unwired: 1 in, 2 out]
          n114 = TCP Read(connection ID=w270, bytes to read=128, 7:T2."Immediate" ("mode (standard)"), 9:w269) -> (data out=→"Error Log":string)  [unwired: 1 in, 2 out]
        }
        event "j1+": Mouse Down {
          n115 = event-data() -> ()  [unwired: 1 in, 8 out]
          n116 = TCP Write(connection ID=w274, data in="MoveJog(j1+)") -> ()  [unwired: 2 in, 3 out]
        }
        event "j2+": Mouse Down {
          n117 = event-data() -> ()  [unwired: 1 in, 8 out]
          n118 = TCP Write(connection ID=w276, data in="MoveJog(j2+)") -> ()  [unwired: 2 in, 3 out]
        }
        event "j3+": Mouse Down {
          n119 = event-data() -> ()  [unwired: 1 in, 8 out]
          n120 = TCP Write(connection ID=w278, data in="MoveJog(j3+)") -> ()  [unwired: 2 in, 3 out]
        }
        event "j4+": Mouse Down {
          n121 = event-data() -> ()  [unwired: 1 in, 8 out]
          n122 = TCP Write(connection ID=w280, data in="MoveJog(j4+)") -> ()  [unwired: 2 in, 3 out]
        }
        event "j5+": Mouse Down {
          n123 = event-data() -> ()  [unwired: 1 in, 8 out]
          n124 = TCP Write(connection ID=w282, data in="MoveJog(j5+)") -> ()  [unwired: 2 in, 3 out]
        }
        event "j6+": Mouse Down {
          n125 = event-data() -> ()  [unwired: 1 in, 8 out]
          n126 = TCP Write(connection ID=w284, data in="MoveJog(j6+)") -> ()  [unwired: 2 in, 3 out]
        }
        event "j1-": Mouse Down {
          n127 = event-data() -> ()  [unwired: 1 in, 8 out]
          n128 = TCP Write(connection ID=w286, data in="MoveJog(j1-)") -> ()  [unwired: 2 in, 3 out]
        }
        event "j2-": Mouse Down {
          n129 = event-data() -> ()  [unwired: 1 in, 8 out]
          n130 = TCP Write(connection ID=w288, data in="MoveJog(j2-)") -> ()  [unwired: 2 in, 3 out]
        }
        event "j3-": Mouse Down {
          n131 = event-data() -> ()  [unwired: 1 in, 8 out]
          n132 = TCP Write(connection ID=w290, data in="MoveJog(j3-)") -> ()  [unwired: 2 in, 3 out]
        }
        event "j4-": Mouse Down {
          n133 = event-data() -> ()  [unwired: 1 in, 8 out]
          n134 = TCP Write(connection ID=w292, data in="MoveJog(j4-)") -> ()  [unwired: 2 in, 3 out]
        }
        event "j5-": Mouse Down {
          n135 = event-data() -> ()  [unwired: 1 in, 8 out]
          n136 = TCP Write(connection ID=w294, data in="MoveJog(j5-)") -> ()  [unwired: 2 in, 3 out]
        }
        event "j6-": Mouse Down {
          n137 = event-data() -> ()  [unwired: 1 in, 8 out]
          n138 = TCP Write(connection ID=w296, data in="MoveJog(j6-)") -> ()  [unwired: 2 in, 3 out]
        }
        event "x+": Mouse Down {
          n139 = event-data() -> ()  [unwired: 1 in, 8 out]
          n140 = TCP Write(connection ID=w298, data in="MoveJog(x+)") -> ()  [unwired: 2 in, 3 out]
        }
        event "y+": Mouse Down {
          n141 = event-data() -> ()  [unwired: 1 in, 8 out]
          n142 = TCP Write(connection ID=w300, data in="MoveJog(y+)") -> ()  [unwired: 2 in, 3 out]
        }
        event "z+": Mouse Down {
          n143 = event-data() -> ()  [unwired: 1 in, 8 out]
          n144 = TCP Write(connection ID=w302, data in="MoveJog(z+)") -> ()  [unwired: 2 in, 3 out]
        }
        event "rx+": Mouse Down {
          n145 = event-data() -> ()  [unwired: 1 in, 8 out]
          n146 = TCP Write(connection ID=w304, data in="MoveJog(rx+)") -> ()  [unwired: 2 in, 3 out]
        }
        event "ry+": Mouse Down {
          n147 = event-data() -> ()  [unwired: 1 in, 8 out]
          n148 = TCP Write(connection ID=w306, data in="MoveJog(ry+)") -> ()  [unwired: 2 in, 3 out]
        }
        event "rz+": Mouse Down {
          n149 = event-data() -> ()  [unwired: 1 in, 8 out]
          n150 = TCP Write(connection ID=w308, data in="MoveJog(rz+)") -> ()  [unwired: 2 in, 3 out]
        }
        event "x-": Mouse Down {
          n151 = event-data() -> ()  [unwired: 1 in, 8 out]
          n152 = TCP Write(connection ID=w310, data in="MoveJog(x-)") -> ()  [unwired: 2 in, 3 out]
        }
        event "y-": Mouse Down {
          n153 = event-data() -> ()  [unwired: 1 in, 8 out]
          n154 = TCP Write(connection ID=w312, data in="MoveJog(y-)") -> ()  [unwired: 2 in, 3 out]
        }
        event "z-": Mouse Down {
          n155 = event-data() -> ()  [unwired: 1 in, 8 out]
          n156 = TCP Write(connection ID=w314, data in="MoveJog(z-)") -> ()  [unwired: 2 in, 3 out]
        }
        event "rx-": Mouse Down {
          n157 = event-data() -> ()  [unwired: 1 in, 8 out]
          n158 = TCP Write(connection ID=w316, data in="MoveJog(rx-)") -> ()  [unwired: 2 in, 3 out]
        }
        event "ry-": Mouse Down {
          n159 = event-data() -> ()  [unwired: 1 in, 8 out]
          n160 = TCP Write(connection ID=w318, data in="MoveJog(ry-)") -> ()  [unwired: 2 in, 3 out]
        }
        event "rz-": Mouse Down {
          n161 = event-data() -> ()  [unwired: 1 in, 8 out]
          n162 = TCP Write(connection ID=w320, data in="MoveJog(rz-)") -> ()  [unwired: 2 in, 3 out]
        }
        event "j6-", "j2+", "j3+", "j4+", "j5+", "j6+", "j1-", "j2-", "j3-", "j4-", "j5-", "x+", "y+", "z+", "rx+", "ry+", "rz+", "x-", "y-", "z-", "rx-", "ry-", "rz-", "j1+": Mouse Up {
          n163 = event-data() -> ()  [unwired: 1 in, 8 out]
          n164 = TCP Write(connection ID=w322, data in="MoveJog()") -> ()  [unwired: 2 in, 3 out]
        }
      }
    }
    n165 = case shown="Default" w15 {
      tunnel: w17 -> [w27 _ w43]
      tunnel: w16 -> [w28 _ w42]
      selector: w15 -> [w29 _ w41]
      frame "EnableRobot()" {
        w35 = "\r\n"
        n166 = local read "Log"() -> (w26:string)
        n167 = TCP Write(connection ID=w28, data in=w29, 9:w27) -> (connection ID out=w36:refnum<k5>)  [unwired: 1 in, 2 out]
        n168 = TCP Read(connection ID=w36, bytes to read=300, 7:T2."Standard" ("mode (standard)"), 9:5000 ("timeout ms (25000)")) -> (data out=w37:string, error out=→"error out 3":errorcluster)  [unwired: 1 in, 1 out]
        n169 = Concatenate Strings(w26, w35, "Send:" ("string"), w29, w35, "Rev:" ("string"), w37) -> (w25:string)
        n170 = local write "Log"(w25) -> ()
      }
      frame "" {
      }
      frame Default {
        w49 = "\r\n"
        n171 = TCP Write(connection ID=w42, data in=w41, 9:w43) -> (connection ID out=w50:refnum<k5>)  [unwired: 1 in, 2 out]
        n172 = local read "Log"() -> (w39:string)
        n173 = TCP Read(connection ID=w50, bytes to read=300, 7:T2."Immediate" ("mode (standard)"), 9:1000 ("timeout ms (25000)")) -> (data out=w51:string, error out=→"error out 2":errorcluster)  [unwired: 1 in, 1 out]
        n174 = Concatenate Strings(w39, w49, "Send:" ("string"), w41, w49, "Rev:" ("string"), w51) -> (w40:string)
        n175 = local write "Log"(w40) -> ()
      }
    }
  }
  n176 = while {
    tunnel: w9 -> [w427]
    tunnel: "stop get state" -> [w424]
    stop <- w423 stop-if-true
    n177 = TCP Read(connection ID=w427, bytes to read=1440, 7:T2."Immediate" ("mode (standard)"), 9:1000 ("timeout ms (25000)")) -> (data out=w425:string, error out=w422:errorcluster)  [unwired: 1 in, 1 out]
    "state error out 2" <- w422
    n178 = String To Byte Array(string=w425) -> (unsigned byte array=w326:u8[])
    n179 = Array Subset(array=w326, index=472, length=8) -> (w341:u8[])
    n180 = Array Subset(array=w326, index=8, length=8) -> (→"DigitalInput":u8[])
    n181 = Array Subset(array=w326, index=448, length=8) -> (w387:u8[])
    n182 = Array Subset(array=w326, index=456, length=8) -> (w385:u8[])
    n183 = Array Subset(array=w326, index=464, length=8) -> (w383:u8[])
    n184 = Array Subset(array=w326, index=440, length=8) -> (w388:u8[])
    n185 = Array Subset(array=w326, index=432, length=8) -> (w391:u8[])
    n186 = Reverse 1D Array(array=w341) -> (reversed array=w340:u8[])
    n187 = Reverse 1D Array(array=w383) -> (reversed array=w382:u8[])
    n188 = Reverse 1D Array(array=w387) -> (reversed array=w386:u8[])
    n189 = Reverse 1D Array(array=w391) -> (reversed array=w390:u8[])
    n190 = Reverse 1D Array(array=w388) -> (reversed array=w389:u8[])
    n191 = Reverse 1D Array(array=w385) -> (reversed array=w384:u8[])
    n192 = Type Cast(type=0.0, x=w340) -> (*(type *) &x=w396:dbl)
    n193 = Type Cast(type=0.0, x=w382) -> (*(type *) &x=w400:dbl)
    n194 = Type Cast(type=0.0, x=w386) -> (*(type *) &x=w408:dbl)
    n195 = Type Cast(type=0.0, x=w389) -> (*(type *) &x=w413:dbl)
    n196 = Type Cast(type=0.0, x=w384) -> (*(type *) &x=w404:dbl)
    n197 = Type Cast(type=0.0, x=w390) -> (*(type *) &x=w418:dbl)
    n198 = Number To Fractional String(number=w396) -> (F-format string=→"j6 value":string)  [unwired: 3 in]
    n199 = Number To Fractional String(number=w408) -> (F-format string=→"j3 value":string)  [unwired: 3 in]
    n200 = Number To Fractional String(number=w404) -> (F-format string=→"j4 value":string)  [unwired: 3 in]
    n201 = Number To Fractional String(number=w400) -> (F-format string=→"j5 value":string)  [unwired: 3 in]
    n202 = Number To Fractional String(number=w413) -> (F-format string=→"j2 value":string)  [unwired: 3 in]
    n203 = Number To Fractional String(number=w418) -> (F-format string=→"j1 value":string)  [unwired: 3 in]
    n204 = Index Array(array=w326, index=24) -> (element=→"Robot mode":u8)
    n205 = Array Subset(array=w326, index=16, length=8) -> (→"DigitalOutput":u8[])
    n206 = Array Subset(array=w326, index=664, length=8) -> (w339:u8[])
    n207 = Array Subset(array=w326, index=640, length=8) -> (w355:u8[])
    n208 = Array Subset(array=w326, index=648, length=8) -> (w353:u8[])
    n209 = Array Subset(array=w326, index=656, length=8) -> (w351:u8[])
    n210 = Array Subset(array=w326, index=632, length=8) -> (w356:u8[])
    n211 = Array Subset(array=w326, index=624, length=8) -> (w343:u8[])
    n212 = Reverse 1D Array(array=w339) -> (reversed array=w338:u8[])
    n213 = Reverse 1D Array(array=w351) -> (reversed array=w350:u8[])
    n214 = Reverse 1D Array(array=w355) -> (reversed array=w354:u8[])
    n215 = Reverse 1D Array(array=w343) -> (reversed array=w342:u8[])
    n216 = Reverse 1D Array(array=w356) -> (reversed array=w357:u8[])
    n217 = Reverse 1D Array(array=w353) -> (reversed array=w352:u8[])
    n218 = Type Cast(type=0.0, x=w338) -> (*(type *) &x=w358:dbl)
    n219 = Type Cast(type=0.0, x=w350) -> (*(type *) &x=w362:dbl)
    n220 = Type Cast(type=0.0, x=w354) -> (*(type *) &x=w370:dbl)
    n221 = Type Cast(type=0.0, x=w357) -> (*(type *) &x=w374:dbl)
    n222 = Type Cast(type=0.0, x=w352) -> (*(type *) &x=w366:dbl)
    n223 = Type Cast(type=0.0, x=w342) -> (*(type *) &x=w378:dbl)
    n224 = Array Subset(array=w326, index=64, length=8) -> (w333:u8[])
    n225 = Number To Fractional String(number=w358) -> (F-format string=→"rz value":string)  [unwired: 3 in]
    n226 = Number To Fractional String(number=w370) -> (F-format string=→"z value":string)  [unwired: 3 in]
    n227 = Number To Fractional String(number=w366) -> (F-format string=→"rx value":string)  [unwired: 3 in]
    n228 = Number To Fractional String(number=w362) -> (F-format string=→"ry value":string)  [unwired: 3 in]
    n229 = Number To Fractional String(number=w374) -> (F-format string=→"y value":string)  [unwired: 3 in]
    n230 = Number To Fractional String(number=w378) -> (F-format string=→"x value":string)  [unwired: 3 in]
    n231 = Reverse 1D Array(array=w333) -> (reversed array=w332:u8[])
    n232 = Type Cast(type=0.0, x=w332) -> (*(type *) &x=→"Current SpeedFactor":dbl)
    n233 = Or(x=w424, y=w422) -> (x .or. y?=w423:bool)
  }
  n234 = TCP Close Connection(connection ID=w13) -> ()  [unwired: 2 in, 2 out]
  n235 = TCP Close Connection(connection ID=w11) -> ()  [unwired: 2 in, 2 out]
  n236 = TCP Close Connection(connection ID=w14) -> ()  [unwired: 2 in, 2 out]
